vi "Tegam4040 - Input Impedance.vi"(0 "Instrument Session Handle In":u32 format="%x", 1 "Input Impedance":enum16{" 1 MOhm", "50 Ohm"}(ring), 11 "error in (no error)":errorcluster) -> (4 "Instrument Session Handle Out (dupl)":u32 format="%x", 15 "error out":errorcluster)   [LabVIEW 2010, in "Tegam4040.lvlib"]
doc: "Input Impedance Mode: This bit select value of impedance mode.\n\n0: 1 MOhm (default)\n1: 50 OHM"
uses:
  Tegam4040.lvlib
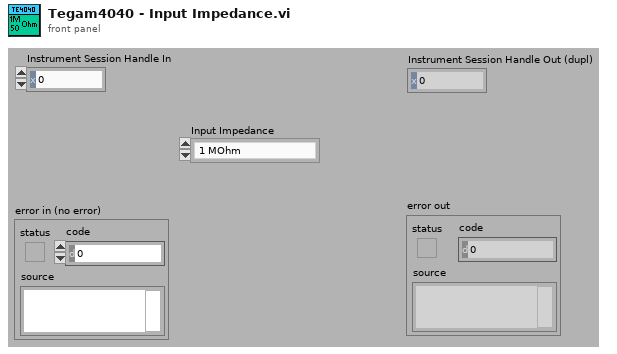
[diagram p1: front panel]
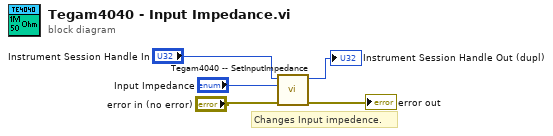
[diagram p0: block diagram]
diagram:
  # "Changes Input impedence."
  n1 = call "Tegam4040 -- SetInputImpedance.vi"("error in (no error)"="error in (no error)", "Input Impedance"="Input Impedance", "Instrument Session Handle In"="Instrument Session Handle In") -> ("error out"=→"error out":errorcluster, "Instrument Session Handle Out (dupl)"=→"Instrument Session Handle Out (dupl)":u32)  [unwired: 7 in]
